vi "ExPlugin_REQUEST_DATA_to_SERVER.vi"(7 "Control Name":string="MOKO_STAGE", 8 "Error In":errorcluster, 11 "MOKO_ExPlugin_STM":T1={"main stm"=enum."idle", "data"="{Hello world!}"}) -> (0 "Error Out":errorcluster)   [LabVIEW 2018]
uses:
  STM/ExPlugin/MOKO_ExPlugin_ExPlugin_STM.ctl
  STM/ExPlugin/MOKO_ExPlugin_ExPlugin_ITEM.ctl
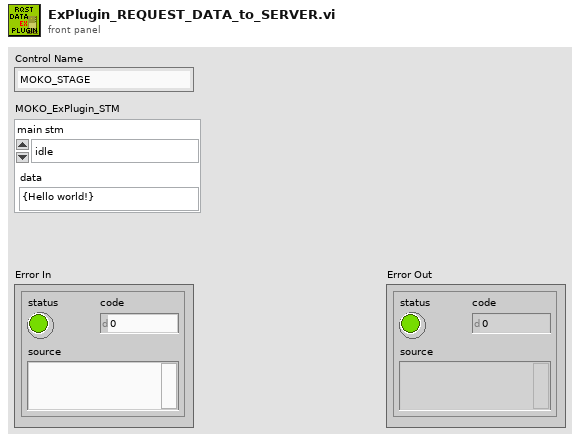
[diagram p1: front panel]
types:
  T1 = typedef "MOKO_ExPlugin_ExPlugin_STM.ctl" = cluster{"main stm":T2, "data":string}
  T2 = typedef "MOKO_ExPlugin_ExPlugin_ITEM.ctl" = enum16{"idle", "ExPlugin read", "ExPlugin write"}
  T3 = enum32{"Invalid", "Default", "Floating", "Floating/Auto-Hide", "Modal"}
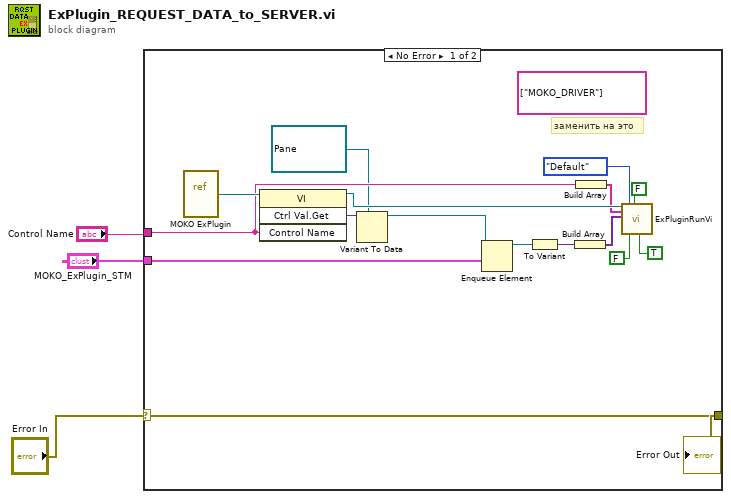
[diagram p0: block diagram]
diagram:
  n1 = case shown="No Error" "Error In" {
    selector: "Error In" -> [w10 w21]
    tunnel: [w10 w21] -> w3
    tunnel: "MOKO_ExPlugin_STM" -> [w9 _]
    tunnel: "Control Name" -> [w8 _]
    frame No Error {
      (unwired) string[] ["MOKO_DRIVER"] ("Controls Name")
      # "заменить на это"
      n2 = vi-ref "MOKO ExPlugin.vi"() -> (w17:refnum<vi>)
      n3 = invoke class="VI" method="Ctrl Val.Get"(reference=w17, "Control Name"=w8) -> (reference out=w20:refnum<vi>, "Get Control Value Variant"=w18:variant)  [unwired: 2 in, 2 out]
      n4 = Variant To Data(type=refnum<queue> refnum ("MOKO_NMEA"), Variant=w18) -> (data=w19:refnum<queue>)  [unwired: 1 in, 1 out]
      n5 = Enqueue Element(queue=w19, element=w9) -> (queue out=w12:refnum<queue>)  [unwired: 2 in, 2 out]
      n6 = To Variant(anything=w12) -> (Variant=w11:variant)
      n7 = Build Array(w11) -> (w16:variant[])
      n8 = Build Array(w8) -> (w7:string[])
      n9 = call "ExPluginRunVi.vi"("VI Refnum"=w20, "Controls Name"=w7, "Values"=w16, "Front Panel Behavior"=T3."Default", "Wait Until Done"=FALSE, "ShowFP"=FALSE, "DoNotCentered If RUN"=TRUE) -> ()  [unwired: 12 in, 1 out]
    }
    frame Error {
    }
  }
  "Error Out" <- w3
